vi "Pre-Build Action.vi"(6 "Top Level/Always Included VIs":path[](array[path]), 7 "Main Destination Path":path, 9 "Target Name":string, 10 "Build Specification Name":string, 11 "Project Path":path) -> (0 "error out":errorcluster)   [LabVIEW 2023]
uses:
  <vilib>/ADAS Replay HIL/AdasReplayUtilities/AdasReplayUtilities.lvlib
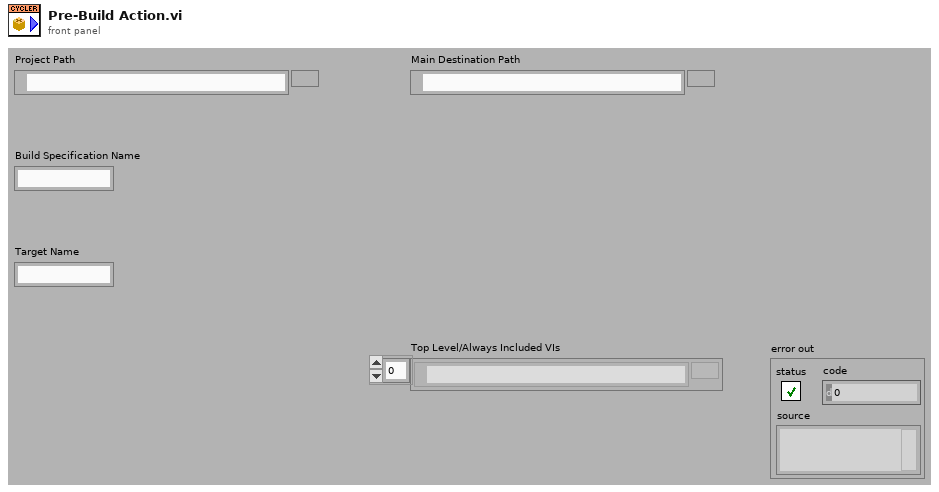
[diagram p1: front panel]
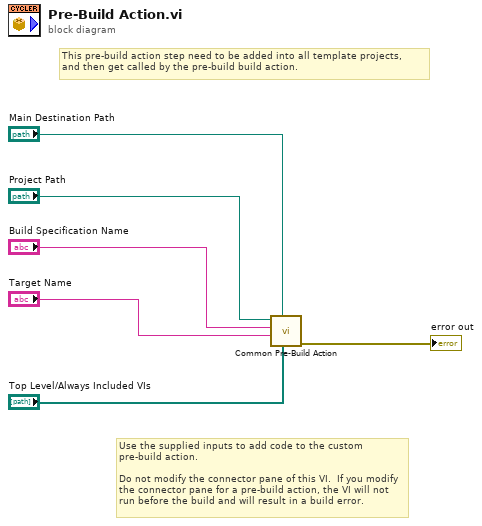
[diagram p0: block diagram]
diagram:
  # "This pre-build action step need to be added into all template projects,\nand then get called by the pre-build build action."
  # "Use the supplied inputs to add code to the custom pre-build action.\n\nDo not modify the connector pane of this VI.  If you modify the connector pane for a pre-build action, the VI will not run before the build and will result in a build error."
  n1 = call <vilib>:"Common Pre-Build Action.vi"("Top Level/Always Included VIs"="Top Level/Always Included VIs", "Main Destination Path"="Main Destination Path", "Target Name"="Target Name", "Build Specification Name"="Build Specification Name", "Project Path"="Project Path") -> ("error out"=→"error out":errorcluster)  [unwired: 6 in]
